vi "Teleop - Reverse Drivebase Orientation.vi"(4 "Reverse Orientation Switch (TB11)":bool, 6 "Normal Orientation Switch (TB10)":bool, 7 "Momentary Flip (TB3)":bool, 8 "In 2":dbl, 11 "In 1":dbl) -> (0 "Out 2":dbl, 3 "Out1":dbl)   [LabVIEW 2015]
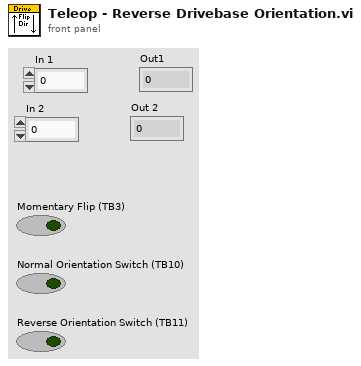
[diagram p1: front panel]
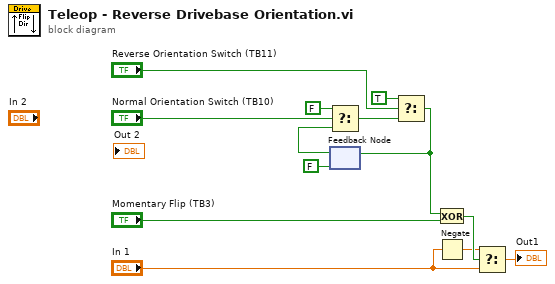
[diagram p0: block diagram]
diagram:
  n1 = feedback #1(FALSE) -> (w2:bool)
  n2 = Select(t=FALSE, s="Normal Orientation Switch (TB10)", f=w2) -> (s? t:f=w3:bool)
  n3 = Select(t=TRUE, s="Reverse Orientation Switch (TB11)", f=w3) -> (s? t:f=w11:bool)
  n4 = feedback-in #1(w11) -> ()
  n5 = Exclusive Or(1:"Momentary Flip (TB3)", 2:w11) -> (0:w13:bool)
  n6 = Negate(x="In 1") -> (-x=w8:dbl)
  n7 = Select(t=w8, s=w13, f="In 1") -> (s? t:f=→"Out1":dbl)
